vi "ADI_IMU_ADIS16448_AHRS_Madgwick.vi"(6 "Yaw Axis":enum16{"X", "Y", "Z"}(ring)=enum."Z", 8 "Reset?":bool, 9 "delta t":dbl, 10 "Beta":dbl, 11 "Data":dbl[](array[numeric])) -> (3 "Output":cluster{"Pitch":dbl, "Roll":dbl, "Yaw":dbl})   [LabVIEW 2019]
uses:
  <vilib>/Analysis/baseanly.llb/Outer Product.vi
  <vilib>/Analysis/baseanly.llb/Real Outer Product.vi
  <vilib>/robotics/Kinematics/Create Lie Group Matrix.vi
  <vilib>/Analysis/coordinate.llb/Direction Cosines To Euler Angles.vi
  <vilib>/Analysis/Matrix/Numeric/Add/Add.vi
  <vilib>/Analysis/Matrix/Numeric/Add/Add - RM,RM.vi
  <vilib>/Analysis/Matrix/Numeric/Multiply/Multiply.vi
  <vilib>/Analysis/Matrix/Numeric/Multiply/Multiply - RM,R.vi
  <vilib>/Analysis/Matrix/Numeric/Multiply/Multiply - R,RM.vi
  <vilib>/robotics/Kinematics/NI_Kinematics.lvlib
panel:
  out "euler angles":T1
  out "Quaternion":dbl[](array[numeric])
  out "Pitch":dbl
  out "Roll":dbl
  out "Yaw":dbl
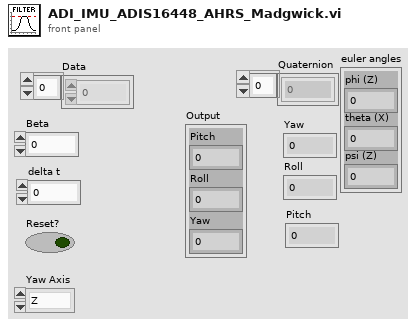
[diagram p1: front panel]
types:
  T1 = cluster{"phi (Z)":dbl, "theta (X)":dbl, "psi (Z)":dbl}
  T2 = typedef "NI_Matrix.lvlib/RealMatrix.ctl" = dbl[][]
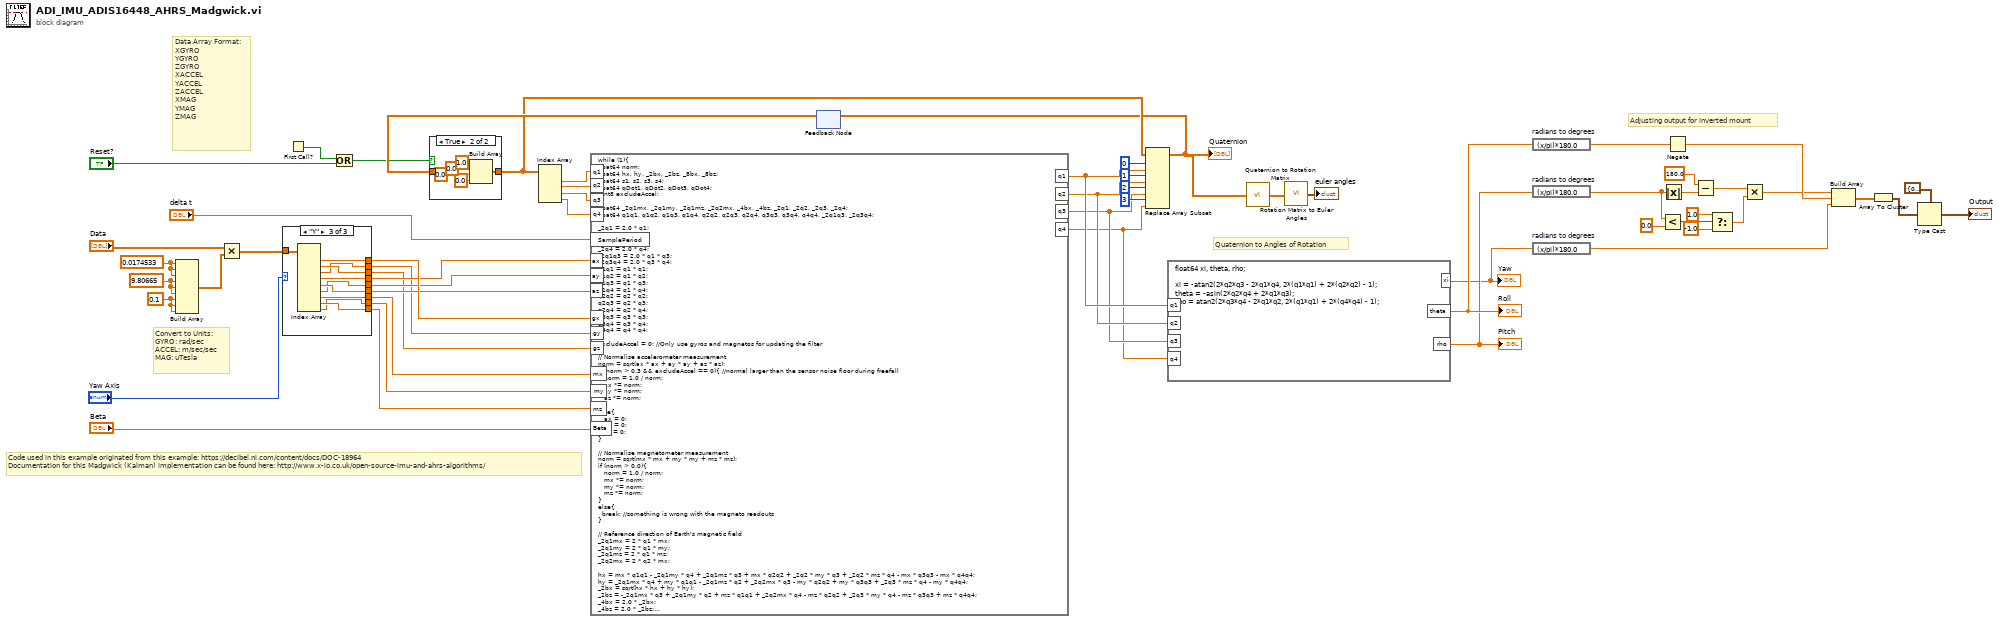
[diagram p0: block diagram]
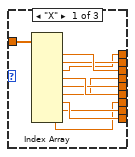
[diagram p2: hidden frame]
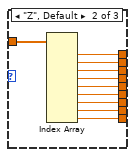
[diagram p3: hidden frame]
diagram:
  w52 = 0.1
  w53 = 9.80665
  w54 = 0.0174533
  # "Code used in this example originated from this example: https://decibel.ni.com/content/docs/DOC-18964\nDocumentation for this Madgwick (Kalman) implementation can be found here: http://www.x-io.co.uk/open-source-imu-and-ahrs-algorithms/"
  # "Quaternion to Angles of Rotation"
  # "Convert to Units:\nGYRO: rad/sec\nACCEL: m/sec/sec\nMAG: uTesla"
  # "Data Array Format:\nXGYRO\nYGYRO\nZGYRO\nXACCEL\nYACCEL\nZACCEL\nXMAG\nYMAG\nZMAG"
  # "Adjusting output for inverted mount"
  n1 = Build Array(w54, w54, w54, w53, w53, w53, w52, w52, w52) -> (w55:dbl[])
  n2 = Multiply(x="Data", y=w55) -> (x*y=w51:dbl[])
  n3 = case shown="\"Y\"" "Yaw Axis" {
    tunnel: [w65 w78 w87] -> w58
    tunnel: [w62 w77 w84] -> w57
    tunnel: w51 -> [w68 w76 w88]
    tunnel: [w59 w75 w81] -> w29
    tunnel: [w63 w74 w82] -> w28
    tunnel: [w64 w73 w83] -> w27
    tunnel: [w66 w72 w85] -> w26
    tunnel: [w67 w71 w86] -> w25
    tunnel: [w60 w70 w79] -> w24
    tunnel: [w61 w69 w80] -> w23
    frame "X" {
      n4 = Index Array(array=w68) -> (element #1=w67:dbl, element #2=w66:dbl, element #3=w65:dbl, element #4=w64:dbl, element #5=w63:dbl, element #6=w62:dbl, element #7=w61:dbl, element #8=w60:dbl, element #9=w59:dbl)  [unwired: 9 in]
    }
    frame "Z", Default {
      n5 = Index Array(array=w76) -> (element #1=w78:dbl, element #2=w72:dbl, element #3=w71:dbl, element #4=w77:dbl, element #5=w74:dbl, element #6=w73:dbl, element #7=w75:dbl, element #8=w70:dbl, element #9=w69:dbl)  [unwired: 9 in]
    }
    frame "Y" {
      n6 = Index Array(array=w88) -> (element #1=w87:dbl, element #2=w86:dbl, element #3=w85:dbl, element #4=w84:dbl, element #5=w83:dbl, element #6=w82:dbl, element #7=w81:dbl, element #8=w80:dbl, element #9=w79:dbl)  [unwired: 9 in]
    }
  }
  n7 = First Call?() -> (First Call?: T/F=w35:bool)
  n8 = Or(x=w35, y="Reset?") -> (x .or. y?=w36:bool)
  n9 = feedback #1() -> (w38:dbl[])  [unwired: 1 in]
  n10 = case shown="True" w36 {
    tunnel: w38 -> [w89 _]
    tunnel: [w89 w90] -> w37
    frame False {
    }
    frame True {
      n11 = Build Array(1.0 ("element"), 0.0 ("element"), 0.0 ("element"), 0.0 ("element")) -> (w90:dbl[])
    }
  }
  n12 = Index Array(array=w37) -> (element #1=w50:dbl, element #2=w49:dbl, element #3=w48:dbl, element #4=w47:dbl)  [unwired: 4 in]
  n13 = formula code="while (1){\nfloat64 norm;\nfloat64 hx, hy, _2bx, _2bz, _8bx, _8bz;\nfloat64 s1, s2, s3, s4;\nfloat64 qDot1, qDot2, qDot3, qDot4;\nuInt8 excludeAccel;\n\nfloat64 _2q1mx, _2q1my, _2q1mz, _2q2mx, _4bx, _4bz, _2q1, _2q2, _2q3, _2q4;\nfloat64 q1q1, q1q2, q1q3, q1q4, q2q2, q2q3, q2q4, q3q3, q3q4, q4q4, _2q1q3, _2q3q4;\n\n_2q1 = 2.0 * q1;\n_2q2 = 2.0 * q2;\n_2q3 = 2.0 * q3;\n_2q4 = 2.0 * q4;\n_2q1q3 = 2.0 * q1 * q3;\n_2q3q4 = 2.0 * q3 * q4;\nq1q1 = q1 * q1;\nq1q2 = q1 * q2;\nq1q3 = q1 * q3;\nq1q4 = q1 * q4;\nq2q2 = q2 * q2;\nq2q3 = q2 * q3;\nq2q4 = q2 * q4;\nq3q3 = q3 * q3;\nq3q4 = q3 * q4;\nq4q4 = q4 * q4;\n\nexcludeAccel = 0; //Only use gyros and magnetos for updating the filter\n\n// Normalise accelerometer measurement\nnorm = sqrt(ax * ax + ay * ay + az * az);\nif (norm > 0.3 && excludeAccel == 0){ //normal larger than the sensor noise floor during freefall\n   norm = 1.0 / norm; \n   ax *= norm;\n   ay *= norm;\n   az *= norm;\n}\nelse{\n   ax = 0;\n   ay = 0;\n   az = 0;\n}\n\n// Normalise magnetometer measurement\nnorm = sqrt(mx * mx + my * my + mz * mz);\nif (norm > 0.0){\n   norm = 1.0 / norm;\n   mx *= norm;\n   my *= norm;\n   mz *= norm;\n}\nelse{\n  break; //something is wrong with the magneto readouts\n}\n\n// Reference direction of Earth's magnetic field\n_2q1mx = 2 * q1 * mx;\n_2q1my = 2 * q1 * my;\n_2q1mz = 2 * q1 * mz;\n_2q2mx = 2 * q2 * mx;\n\nhx = mx * q1q1 - _2q1my * q4 + _2q1mz * q3 + mx * q2q2 + _2q2 * my * q3 + _2q2 * mz * q4 - mx * q3q3 - mx * q4q4;\nhy = _2q1mx * q4 + my * q1q1 - _2q1mz * q2 + _2q2mx * q3 - my * q2q2 + my * q3q3 + _2q3 * mz * q4 - my * q4q4;\n_2bx = sqrt(hx * hx + hy * hy);\n_2bz = -_2q1mx * q3 + _2q1my * q2 + mz * q1q1 + _2q2mx * q4 - mz * q2q2 + _2q3 * my * q4 - mz * q3q3 + mz * q4q4;\n_4bx = 2.0 * _2bx;\n_4bz = 2.0 * _2bz;\n_8bx = 2.0 * _4bx;\n_8bz = 2.0 * _4bz;\n\n// Gradient descent algorithm corrective step\ns1 = -_2q3 * (2.0 * q2q4 - _2q1q3 - ax) + _2q2 * (2.0 * q1q2 + _2q3q4 - ay) - _4bz * q3 * (_4bx * (0.5 - q3q3 - q4q4) + _4bz * (q2q4 - q1q3) - mx) + (-_4bx * q4 + _4bz * q2) * (_4bx * (q2q3 - q1q4) + _4bz * (q1q2 + q3q4) - my) + _4bx * q3 * (_4bx * (q1q3 + q2q4) + _4bz * (0.5 - q2q2 - q3q3) - mz);\ns2 = _2q4 * (2.0 * q2q4 - _2q1q3 - ax) + _2q1 * (2.0 * q1q2 + _2q3q4 - ay) - 4.0 * q2 * (1.0 - 2.0 * q2q2 - 2.0 * q3q3 - az) + _4bz * q4 * (_4bx * (0.5 - q3q3 - q4q4) + _4bz * (q2q4 - q1q3) - mx) + (_4bx * q3 + _4bz * q1) * (_4bx * (q2q3 - q1q4) + _4bz * (q1q2 + q3q4) - my) + (_4bx * q4 - _8bz * q2) * (_4bx * (q1q3 + q2q4) + _4bz * (0.5 - q2q2 - q3q3) - mz);\ns3 = -_2q1 * (2.0 * q2q4 - _2q1q3 - ax) + _2q4 * (2.0 * q1q2 + _2q3q4 - ay) - 4.0 * q3 * (1.0 - 2.0 * q2q2 - 2.0 * q3q3 - az) + (-_8bx * q3 - _4bz * q1) * (_4bx * (0.5 - q3q3 - q4q4) + _4bz * (q2q4 - q1q3) - mx) + (_4bx * q2 + _4bz * q4) * (_4bx * (q2q3 - q1q4) + _4bz * (q1q2 + q3q4) - my) + (_4bx * q1 - _8bz * q3) * (_4bx * (q1q3 + q2q4) + _4bz * (0.5 - q2q2 - q3q3) - mz);\ns4 = _2q2 * (2.0 * q2q4 - _2q1q3 - ax) + _2q3 * (2.0 * q1q2 + _2q3q4 - ay) + (-_8bx * q4 + _4bz * q2) * (_4bx * (0.5 - q3q3 - q4q4) + _4bz * (q2q4 - q1q3) - mx) + (-_4bx * q1 + _4bz * q3) * (_4bx * (q2q3 - q1q4) + _4bz * (q1q2 + q3q4) - my) + _4bx * q2 * (_4bx * (q1q3 + q2q4) + _4bz * (0.5 - q2q2 - q3q3) - mz);\n\nnorm = sqrt(s1 * s1 + s2 * s2 + s3 * s3 + s4 * s4);\nif (norm > 0.0){\n   norm = 1.0 / norm;  //normalise gradient step\n   s1 *= norm;\n   s2 *= norm;\n   s3 *= norm;\n   s4 *= norm;\n}\nelse{\n   break;\n}\n\n// Compute rate of change of quaternion\nqDot1 = 0.5 * (-q2 * gx - q3 * gy - q4 * gz) - Beta * s1;\nqDot2 = 0.5 * (q1 * gx + q3 * gz - q4 * gy) - Beta * s2;\nqDot3 = 0.5 * (q1 * gy - q2 * gz + q4 * gx) - Beta * s3;\nqDot4 = 0.5 * (q1 * gz + q2 * gy - q3 * gx) - Beta * s4;\n\n// Integrate to yield quaternion\nq1 += qDot1 * SamplePeriod;\nq2 += qDot2 * SamplePeriod;\nq3 += qDot3 * SamplePeriod;\nq4 += qDot4 * SamplePeriod;\n\nnorm = sqrt(q1 * q1 + q2 * q2 + q3 * q3 + q4 * q4);\nif (norm > 0.0){\n   norm = 1.0 / norm;  //normalise quaternion\n   q1 = q1 * norm;\n   q2 = q2 * norm;\n   q3 = q3 * norm;\n   q4 = q4 * norm;\n}\nbreak;\n}"("q1"=w50, "gx"=w58, "gy"=w26, "gz"=w25, "ax"=w57, "ay"=w28, "az"=w27, "mx"=w29, "my"=w24, "mz"=w23, "SamplePeriod"="delta t", "Beta"="Beta", "q2"=w49, "q3"=w48, "q4"=w47) -> ("q1"=w42:dbl, "q2"=w41:dbl, "q3"=w40:dbl, "q4"=w39:dbl)
  n14 = Replace Array Subset(array=w37, new element #1=w42, index #1=0 ("index"), new element #2=w41, index #2=1 ("index"), new element #3=w40, index #3=2 ("index"), new element #4=w39, index #4=3 ("index")) -> (w2:dbl[])
  "Quaternion" <- w2
  n15 = feedback-in #1(w2) -> ()
  n16 = formula code="float64 xi, theta, rho;\n\nxi = -atan2(2*q2*q3 - 2*q1*q4, 2*(q1*q1) + 2*(q2*q2) - 1);\ntheta = -asin(2*q2*q4 + 2*q1*q3);\nrho = atan2(2*q3*q4 - 2*q1*q2, 2*(q1*q1) + 2*(q4*q4) - 1);"("q1"=w42, "q2"=w41, "q3"=w40, "q4"=w39) -> ("xi"=w31:dbl, "theta"=w33:dbl, "rho"=w32:dbl)
  "Yaw" <- w31
  "Roll" <- w33
  "Pitch" <- w32
  n17 = call <vilib>:"Quaternion to Rotation Matrix.vi"("quaternion"=w2) -> ("rotation matrix"=w3:T2)
  n18 = call <vilib>:"Rotation Matrix to Euler Angles.vi"("rotation matrix"=w3) -> ("euler angles"=→"euler angles":T1)
  n19 = expression code="(x/pi)*180.0" "radians to degrees"(w33) -> (w13:dbl)
  n20 = expression code="(x/pi)*180.0" "radians to degrees"(w32) -> (w20:dbl)
  n21 = expression code="(x/pi)*180.0" "radians to degrees"(w31) -> (w30:dbl)
  n22 = Less?(x=w20, y=0.0) -> (x < y?=w18:bool)
  n23 = Absolute Value(x=w20) -> (abs(x)=w22:dbl)
  n24 = Negate(x=w13) -> (-x=w12:dbl)
  n25 = Subtract(x=180.0 ("y"), y=w22) -> (x-y=w15:dbl)
  n26 = Select(t=1.0, s=w18, f=-1.0) -> (s? t:f=w14:dbl)
  n27 = Multiply(x=w15, y=w14) -> (x*y=w11:dbl)
  n28 = Build Array(w11, w12, w30) -> (w6:dbl[])
  n29 = Array To Cluster(array=w6) -> (cluster=w7:cluster{"[0]":dbl, "[1]":dbl, "[2]":dbl})
  n30 = Type Cast(type=cluster{"Pitch":dbl, "Roll":dbl, "Yaw":dbl} {"Pitch"=0.0, "Roll"=0.0, "Yaw"=0.0} ("IMU AHRS"), x=w7) -> (*(type *) &x=→"Output":cluster{"Pitch":dbl, "Roll":dbl, "Yaw":dbl})
